vi "Set All Values.vi"(10 "Values":T1, 11 "User in":refnum<class "User.lvclass">) -> (0 "error out":errorcluster, 3 "User out":refnum<class "User.lvclass">)   [LabVIEW 2020, in "Test.lvlib" / "User.lvclass"]
uses:
  User.lvclass
  <vilib>/IlluminatedG/IG Conditum/Conditum/Columns/Boolean/Boolean.lvclass
  <vilib>/IlluminatedG/IG Conditum/Conditum/Columns/Integer/Integer.lvclass
  <vilib>/IlluminatedG/IG Conditum/Conditum/Columns/String/String.lvclass
  <vilib>/IlluminatedG/IG Conditum/Conditum/Columns/Timestamp/Timestamp.lvclass
  Values.ctl
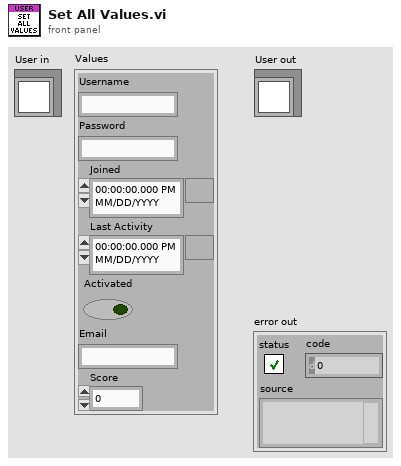
[diagram p1: front panel]
types:
  T1 = typedef "Test.lvlib/User.lvclass/Values.ctl" = cluster{"Username":string, "Password":string, "Joined":timestamp, "Last Activity":timestamp, "Activated":bool, "Email":string, "Score":i64}
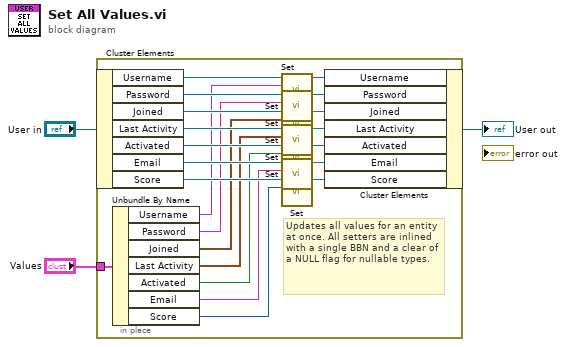
[diagram p0: block diagram]
diagram:
  n1 = in-place {
    in-place-border: "Values" -> [w18]
    # "Updates all values for an entity at once. All setters are inlined with a single BBN and a clear of a NULL flag for nullable types."
    n2 = in-place-cluster #1("User in") -> ("Username"=w25:refnum<class "String.lvclass">, "Password"=w24:refnum<class "String.lvclass">, "Joined"=w23:refnum<class "Timestamp.lvclass">, "Last Activity"=w22:refnum<class "Timestamp.lvclass">, "Activated"=w21:refnum<class "Boolean.lvclass">, "Email"=w20:refnum<class "String.lvclass">, "Score"=w19:refnum<class "Integer.lvclass">)
    n3 = Unbundle By Name(w18) -> ("Username"=w17:string, "Password"=w16:string, "Joined"=w15:timestamp, "Last Activity"=w14:timestamp, "Activated"=w13:bool, "Email"=w12:string, "Score"=w11:i64)
    n4 = call <vilib>:"Set.vi"("Value"=w17, "String in"=w25) -> ("String out"=w4:refnum<class "String.lvclass">)  [unwired: 9 in]
    n5 = call <vilib>:"Set.vi"("Value"=w16, "String in"=w24) -> ("String out"=w5:refnum<class "String.lvclass">)  [unwired: 9 in]
    n6 = call <vilib>:"Set.vi"("Time Stamp"=w15, "DateTime in"=w23) -> ("DateTime out"=w6:refnum<class "Timestamp.lvclass">)  [unwired: 9 in]
    n7 = call <vilib>:"Set.vi"("Time Stamp"=w14, "DateTime in"=w22) -> ("DateTime out"=w7:refnum<class "Timestamp.lvclass">)  [unwired: 9 in]
    n8 = call <vilib>:"Set.vi"("Value"=w13, "Boolean in"=w21) -> ("Boolean out"=w8:refnum<class "Boolean.lvclass">)  [unwired: 9 in]
    n9 = call <vilib>:"Set.vi"("Value"=w12, "String in"=w20) -> ("String out"=w9:refnum<class "String.lvclass">)  [unwired: 9 in]
    n10 = call <vilib>:"Set.vi"("Value"=w11, "Integer in"=w19) -> ("Integer out"=w10:refnum<class "Integer.lvclass">)  [unwired: 9 in]
    n11 = in-place-cluster #1("Username"=w4, "Password"=w5, "Joined"=w6, "Last Activity"=w7, "Activated"=w8, "Email"=w9, "Score"=w10) -> (→"User out":refnum<class "User.lvclass">)
  }
